vi "Read Modes.vi"(8 "error in (no error)":errorcluster, 11 "Template in":refnum<class "MetaDataObj.lvclass">) -> (0 "error out":errorcluster, 2 "Modes":string[](array[string]), 3 "Template out":refnum<class "MetaDataObj.lvclass">)   [LabVIEW 2016, in "MetaDataObj.lvclass"]
uses:
  <resource>/dialog/NewProjectWizard/MetaDataObj/MetaDataObj.lvclass
  <resource>/dialog/NewProjectWizard/MetaDataObj/MetaDataObj.lvclass/MetaDataObj.ctl
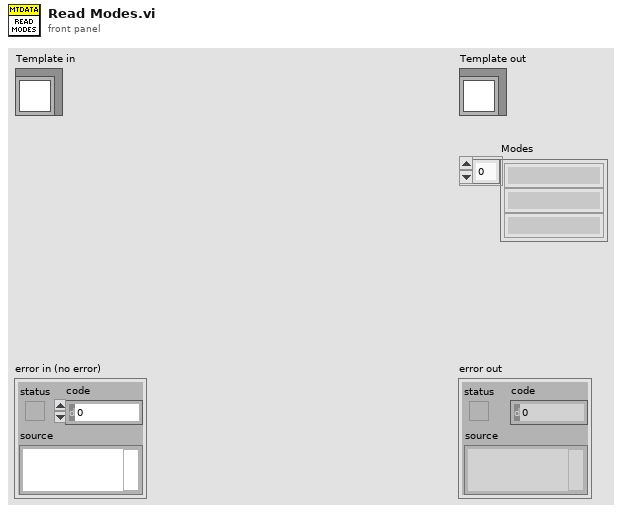
[diagram p1: front panel]
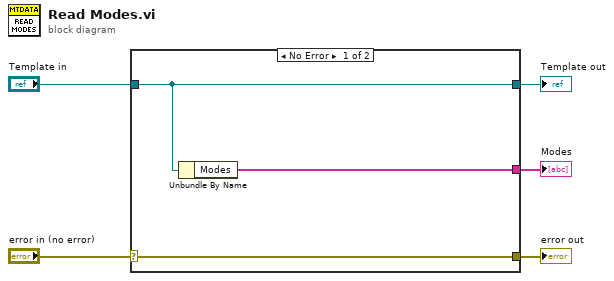
[diagram p0: block diagram]
diagram:
  n1 = case shown="No Error" "error in (no error)" {
    selector: "error in (no error)" -> [w8 w9]
    tunnel: [w8 w9] -> w4
    tunnel: [w7 w10] -> w2
    tunnel: "Template in" -> [w7 w10]
    tunnel: [w6 _] -> w1
    frame No Error {
      n2 = Unbundle By Name(w7) -> ("Modes"=w6:string[])
    }
    frame Error {
    }
  }
  "error out" <- w4
  "Template out" <- w2
  "Modes" <- w1
